vi "TestActuator.vi"(3 "Input_Value_Boolean":bool, 4 "Input_Value_Double":dbl, 5 "Actuator_Name":string) -> (0 "Output_Value_Boolean":bool, 1 "Output_Value_Double":dbl, 2 "In_Test_Mode":bool)   [LabVIEW 2019]
uses:
  dsdata.vi
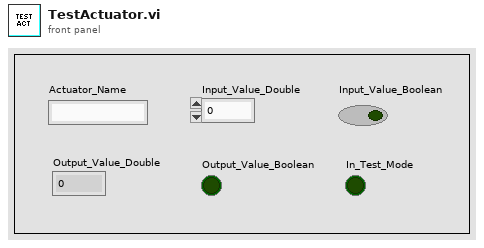
[diagram p1: front panel]
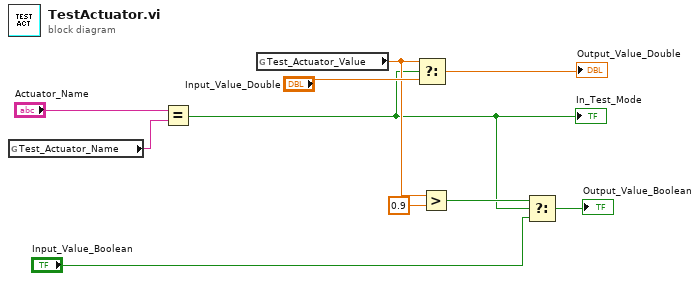
[diagram p0: block diagram]
diagram:
  n1 = global read "dsdata.vi" "Test_Actuator_Name"() -> (w8:string)
  n2 = Equal?(x="Actuator_Name", y=w8) -> (x = y?=w1:bool)
  "In_Test_Mode" <- w1
  n3 = global read "dsdata.vi" "Test_Actuator_Value"() -> (w6:dbl)
  n4 = Select(t=w6, s=w1, f="Input_Value_Double") -> (s? t:f=→"Output_Value_Double":dbl)
  n5 = Greater?(x=w6, y=0.9) -> (0:w4:bool)
  n6 = Select(t=w4, s=w1, f="Input_Value_Boolean") -> (s? t:f=→"Output_Value_Boolean":bool)
